vi "Init.vi"(8 "error in (no error)":errorcluster, 11 "Data in":refnum<class "Local Bus.lvclass">) -> (0 "error out":errorcluster, 3 "Data out":refnum<class "Local Bus.lvclass">)   [LabVIEW 2021, in "Local Bus.lvclass"]
uses:
  Local Bus.lvclass
  C:/TSA/Omni-Bus/Source/Omni-Bus/Bus Access/Bus_Access.lvclass
  Support/Type Counts.ctl
  Local Bus.lvclass/Local Bus.ctl
  Support/Type/Local Bus_Type.lvclass
  C:/Program Files (x86)/National Instruments/LabVIEW 2021/vi.lib/TSA/Abstract Data Classes/Abs_Types/Type/Abs_Type.lvclass
  Support/DBL/Local Bus_DBL.lvclass
  C:/Program Files (x86)/National Instruments/LabVIEW 2021/vi.lib/TSA/Abstract Data Classes/Abs_Types/Value/Abs_Value.lvclass
  Support/SGL/Local Bus_SGL.lvclass
  Support/EXT/Local Bus_EXT.lvclass
  Support/Bool/Local Bus_Boolean.lvclass
  Support/STR/Local Bus_String.lvclass
  Support/Variant/Local Bus_Variant.lvclass
  Support/WFM/Local Bus_Waveform.lvclass
  Support/Time/Local Bus_Time.lvclass
  Support/U8/Local Bus_U8.lvclass
  Support/U16/Local Bus_U16.lvclass
  Support/U32/Local Bus_U32.lvclass
  Support/U64/Local Bus_U64.lvclass
  Support/I8/Local Bus_I8.lvclass
  Support/I16/Local Bus_I16.lvclass
  Support/I32/Local Bus_I32.lvclass
  Support/I64/Local Bus_I64.lvclass
  Support/CSGL/Local Bus_CSGL.lvclass
  Support/CDBL/Local Bus_CDBL.lvclass
  Support/CEXT/Local Bus_CEXT.lvclass
  Omni-Bus/Bus Access/Bus_Access.lvclass/Bus_Access.ctl
  Properties/Read Tag Types.vi
  Properties/Read Initial Values.vi
  Omni-Bus/Bus Access/Properties/Write Values.vi
  <vilib>/TSA/Abstract Data Classes/Abs_Types/Value/Abs_Value.lvclass
  <vilib>/Utility/error.llb/Error Cluster From Error Code.vi
  <vilib>/ErrorRing/Error Ring.xnode
  Omni-Bus/Bus Access/Bus_Access.lvclass
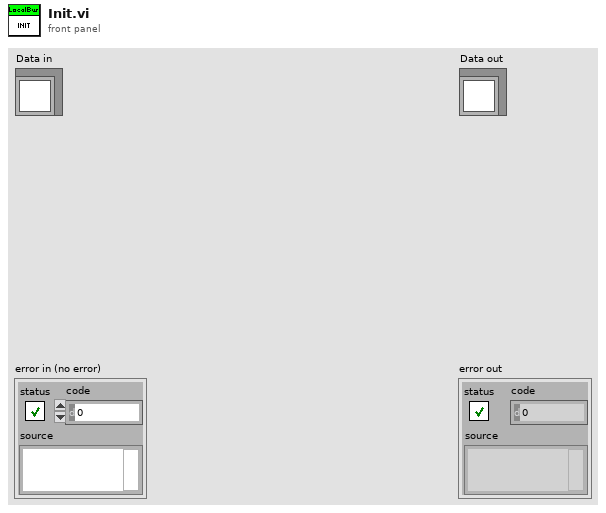
[diagram p1: front panel]
types:
  T1 = typedef "Local Bus.lvclass/Type Counts.ctl" = cluster{"Boolean":i32, "String":i32, "DBL":i32, "SGL":i32, "EXT":i32, "U8":i32, "U16":i32, "U32":i32, "U64":i32, "I8":i32, "I16":i32, "I32":i32, "I64":i32, "CDBL":i32, "CSGL":i32, "CEXT":i32, "Time":i32, "Variant":i32, "Waveform":i32, "Object":i32}
  T2 = typedef "NI_Data Type.lvlib/Data Type.ctl" = enum8{"Invalid Type", "Void", "I8", "I16", "I32", "I64", "U8", "U16", "U32", "U64", "Single Float", "Double Float", "Extended Float", "Single Complex", "Double Complex", "Extended Complex", "Enum U8", "Enum U16", "Enum U32", "Enum U64", "Single Float With Unit", "Double Float With Unit", "Extended Float With Unit", "Single Complex with Unit", "Double Complex with Unit", "Extended Complex with Unit", "Boolean", "String", "Path", "Picture", "Tag", "Array", "Cluster", "Variant", "LV Variant", "Waveform", "Timestamp", "Digital Waveform", "Digital Data", "ExpressData", "Refnum", "External Data", "VI", "Poly VI", "LabVIEW Class Instance", "Fixed Point", "Set Collection", "Map Collection"}
  T3 = typedef "Local Bus.lvclass/Data Value References.ctl" = cluster{"Boolean":refnum<data-value>, "String":refnum<data-value>, "DBL":refnum<data-value>, "SGL":refnum<data-value>, "EXT":refnum<data-value>, "U8":refnum<data-value>, "U16":refnum<data-value>, "U32":refnum<data-value>, "U64":refnum<data-value>, "I8":refnum<data-value>, "I16":refnum<data-value>, "I32":refnum<data-value>, "I64":refnum<data-value>, "CDBL":refnum<data-value>, "CSGL":refnum<data-value>, "CEXT":refnum<data-value>, "Time":refnum<data-value>, "Variant":refnum<data-value>, "Waveform":refnum<data-value>, "Type":refnum<data-value>}
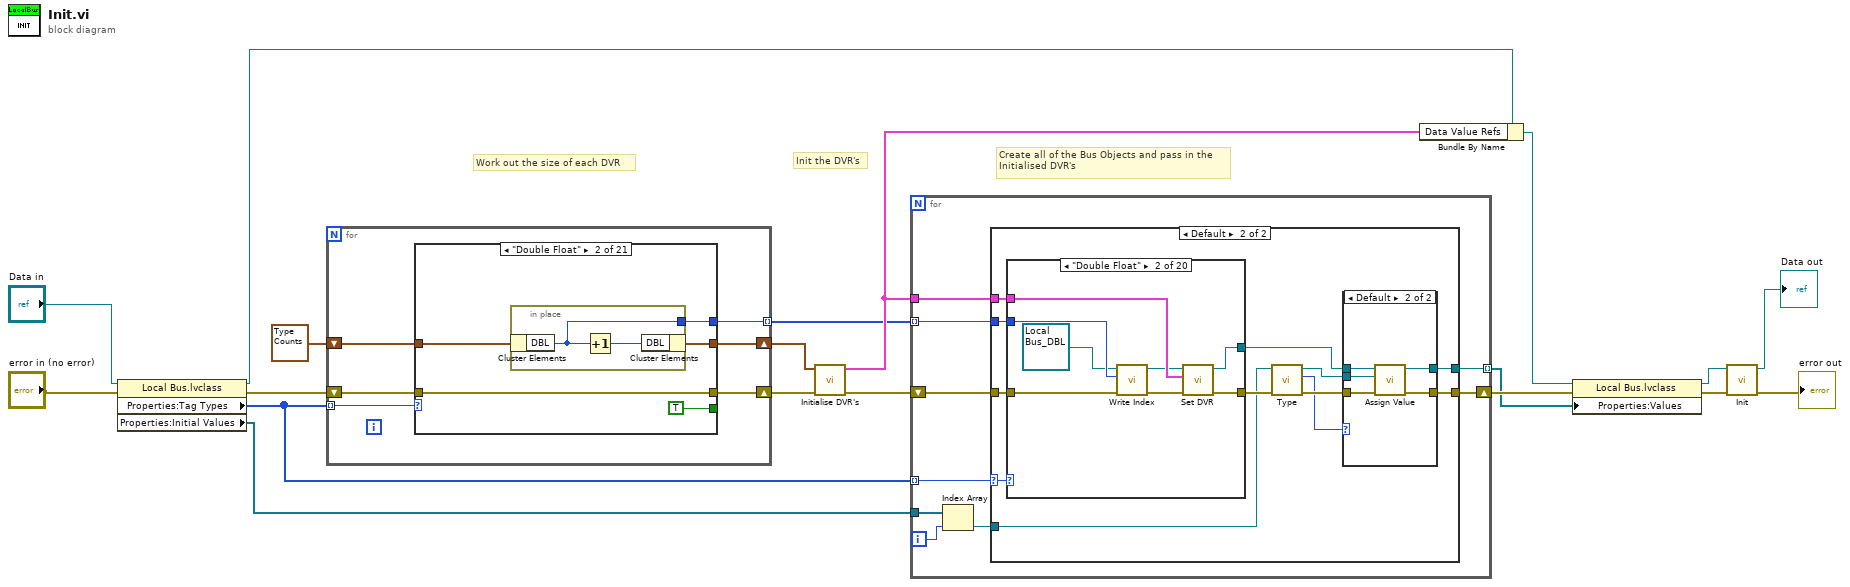
[diagram p0: block diagram]
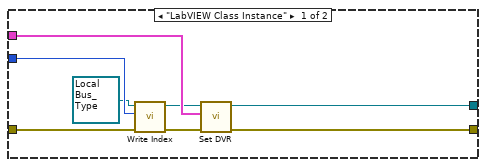
[diagram p2: hidden frame]
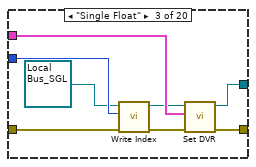
[diagram p5: hidden frame]
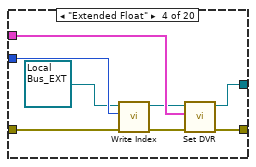
[diagram p6: hidden frame]
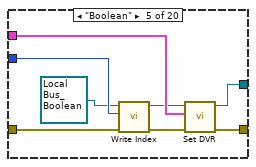
[diagram p7: hidden frame]
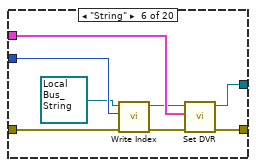
[diagram p8: hidden frame]
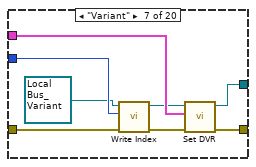
[diagram p9: hidden frame]
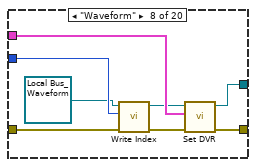
[diagram p10: hidden frame]
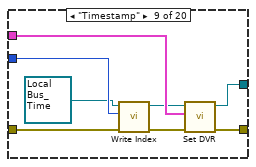
[diagram p11: hidden frame]
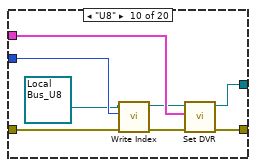
[diagram p12: hidden frame]
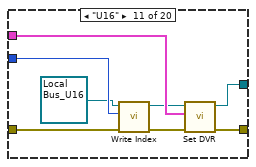
[diagram p13: hidden frame]
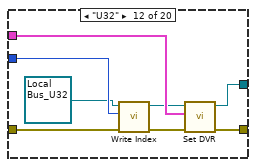
[diagram p14: hidden frame]
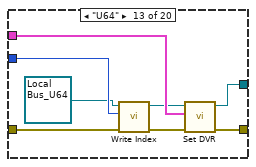
[diagram p15: hidden frame]
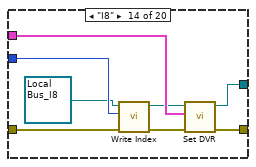
[diagram p16: hidden frame]
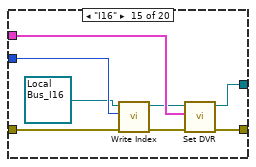
[diagram p17: hidden frame]
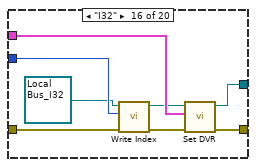
[diagram p18: hidden frame]
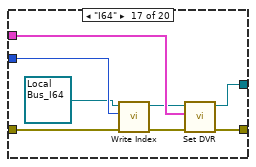
[diagram p19: hidden frame]
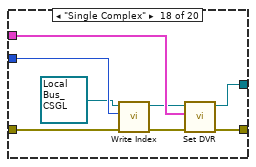
[diagram p20: hidden frame]
diagram:
  # "Create all of the Bus Objects and pass in the\nInitialised DVR's"
  # "Init the DVR's"
  # "Work out the size of each DVR"
  n1 = property class="Local Bus.lvclass"(reference="Data in", error in="error in (no error)") -> (reference out=w16:refnum<class "Local Bus.lvclass">, error out=w17:errorcluster, "Properties:Tag Types"=w6:T2[], "Properties:Initial Values"=w5:refnum<class "Abs_Value.lvclass">[])
  n2 = for {
    shift-right: [w22] -> w14
    shift-left: w17 -> [w25]
    shift-right: [w23] -> w13
    shift-left: T1 {"Boolean"=0, "String"=0, "DBL"=0, "SGL"=0, "EXT"=0, "U8"=0, "U16"=0, "U32"=0, "U64"=0, "I8"=0, "I16"=0, "I32"=0, "I64"=0, "CDBL"=0, "CSGL"=0, "CEXT"=0, "Time"=0, "Variant"=0, "Waveform"=0, "Object"=0} ("Type Counts") -> [w24]
    tunnel: [w21] -> w7 mode=indexing
    tunnel: w6 -> [w20] mode=indexing
    n3 = case shown="\"Double Float\"" w20 {
      tunnel: w25 -> [_ w38 w45 w52 w59 w66 w73 w80 w87 w94 w101 w108 w115 w122 w129 w136 w143 w150 w157 w164 w171]
      tunnel: w24 -> [w28 w37 w44 w51 w58 w65 w72 w79 w86 w93 w100 w107 w114 w121 w128 w135 w142 w149 w156 w163 w170]
      tunnel: [w28 w36 w43 w50 w57 w64 w71 w78 w85 w92 w99 w106 w113 w120 w127 w134 w141 w148 w155 w162 w169] -> w23
      tunnel: [w26 w38 w45 w52 w59 w66 w73 w80 w87 w94 w101 w108 w115 w122 w129 w136 w143 w150 w157 w164 w171] -> w22
      tunnel: [FALSE TRUE TRUE TRUE TRUE TRUE TRUE TRUE TRUE TRUE TRUE TRUE TRUE TRUE TRUE TRUE TRUE TRUE TRUE TRUE TRUE] -> _
      tunnel: [_ w34 w41 w48 w55 w62 w69 w76 w83 w90 w97 w104 w111 w118 w125 w132 w139 w146 w153 w160 w167] -> w21
      frame "Invalid Type", Default {
        n4 = xnode "Error Ring"() -> ("error out"=w26:errorcluster)
      }
      frame "Double Float" {
        n5 = in-place {
          in-place-border: [w39] -> w34
          n6 = in-place-cluster #1(w37) -> ("DBL"=w39:i32)
          n7 = Increment(x=w39) -> (x+1=w40:i32)
          n8 = in-place-cluster #1("DBL"=w40) -> (w36:T1)
        }
      }
      frame "Single Float" {
        n9 = in-place {
          in-place-border: [w46] -> w41
          n10 = in-place-cluster #2(w44) -> ("SGL"=w46:i32)
          n11 = Increment(x=w46) -> (x+1=w47:i32)
          n12 = in-place-cluster #2("SGL"=w47) -> (w43:T1)
        }
      }
      frame "Extended Float" {
        n13 = in-place {
          in-place-border: [w53] -> w48
          n14 = in-place-cluster #3(w51) -> ("EXT"=w53:i32)
          n15 = Increment(x=w53) -> (x+1=w54:i32)
          n16 = in-place-cluster #3("EXT"=w54) -> (w50:T1)
        }
      }
      frame "Boolean" {
        n17 = in-place {
          in-place-border: [w60] -> w55
          n18 = in-place-cluster #4(w58) -> ("Boolean"=w60:i32)
          n19 = Increment(x=w60) -> (x+1=w61:i32)
          n20 = in-place-cluster #4("Boolean"=w61) -> (w57:T1)
        }
      }
      frame "String" {
        n21 = in-place {
          in-place-border: [w67] -> w62
          n22 = in-place-cluster #5(w65) -> ("String"=w67:i32)
          n23 = Increment(x=w67) -> (x+1=w68:i32)
          n24 = in-place-cluster #5("String"=w68) -> (w64:T1)
        }
      }
      frame "Waveform" {
        n25 = in-place {
          in-place-border: [w74] -> w69
          n26 = in-place-cluster #6(w72) -> ("Waveform"=w74:i32)
          n27 = Increment(x=w74) -> (x+1=w75:i32)
          n28 = in-place-cluster #6("Waveform"=w75) -> (w71:T1)
        }
      }
      frame "Timestamp" {
        n29 = in-place {
          in-place-border: [w81] -> w76
          n30 = in-place-cluster #7(w79) -> ("Time"=w81:i32)
          n31 = Increment(x=w81) -> (x+1=w82:i32)
          n32 = in-place-cluster #7("Time"=w82) -> (w78:T1)
        }
      }
      frame "Variant" {
        n33 = in-place {
          in-place-border: [w88] -> w83
          n34 = in-place-cluster #8(w86) -> ("Variant"=w88:i32)
          n35 = Increment(x=w88) -> (x+1=w89:i32)
          n36 = in-place-cluster #8("Variant"=w89) -> (w85:T1)
        }
      }
      frame "LabVIEW Class Instance" {
        n37 = in-place {
          in-place-border: [w95] -> w90
          n38 = in-place-cluster #9(w93) -> ("Object"=w95:i32)
          n39 = Increment(x=w95) -> (x+1=w96:i32)
          n40 = in-place-cluster #9("Object"=w96) -> (w92:T1)
        }
      }
      frame "U8" {
        n41 = in-place {
          in-place-border: [w102] -> w97
          n42 = in-place-cluster #10(w100) -> ("U8"=w102:i32)
          n43 = Increment(x=w102) -> (x+1=w103:i32)
          n44 = in-place-cluster #10("U8"=w103) -> (w99:T1)
        }
      }
      frame "U16" {
        n45 = in-place {
          in-place-border: [w109] -> w104
          n46 = in-place-cluster #11(w107) -> ("U16"=w109:i32)
          n47 = Increment(x=w109) -> (x+1=w110:i32)
          n48 = in-place-cluster #11("U16"=w110) -> (w106:T1)
        }
      }
      frame "U32" {
        n49 = in-place {
          in-place-border: [w116] -> w111
          n50 = in-place-cluster #12(w114) -> ("U32"=w116:i32)
          n51 = Increment(x=w116) -> (x+1=w117:i32)
          n52 = in-place-cluster #12("U32"=w117) -> (w113:T1)
        }
      }
      frame "U64" {
        n53 = in-place {
          in-place-border: [w123] -> w118
          n54 = in-place-cluster #13(w121) -> ("U64"=w123:i32)
          n55 = Increment(x=w123) -> (x+1=w124:i32)
          n56 = in-place-cluster #13("U64"=w124) -> (w120:T1)
        }
      }
      frame "I8" {
        n57 = in-place {
          in-place-border: [w130] -> w125
          n58 = in-place-cluster #14(w128) -> ("I8"=w130:i32)
          n59 = Increment(x=w130) -> (x+1=w131:i32)
          n60 = in-place-cluster #14("I8"=w131) -> (w127:T1)
        }
      }
      frame "I16" {
        n61 = in-place {
          in-place-border: [w137] -> w132
          n62 = in-place-cluster #15(w135) -> ("I16"=w137:i32)
          n63 = Increment(x=w137) -> (x+1=w138:i32)
          n64 = in-place-cluster #15("I16"=w138) -> (w134:T1)
        }
      }
      frame "I32" {
        n65 = in-place {
          in-place-border: [w144] -> w139
          n66 = in-place-cluster #16(w142) -> ("I32"=w144:i32)
          n67 = Increment(x=w144) -> (x+1=w145:i32)
          n68 = in-place-cluster #16("I32"=w145) -> (w141:T1)
        }
      }
      frame "I64" {
        n69 = in-place {
          in-place-border: [w151] -> w146
          n70 = in-place-cluster #17(w149) -> ("I64"=w151:i32)
          n71 = Increment(x=w151) -> (x+1=w152:i32)
          n72 = in-place-cluster #17("I64"=w152) -> (w148:T1)
        }
      }
      frame "Single Complex" {
        n73 = in-place {
          in-place-border: [w158] -> w153
          n74 = in-place-cluster #18(w156) -> ("CSGL"=w158:i32)
          n75 = Increment(x=w158) -> (x+1=w159:i32)
          n76 = in-place-cluster #18("CSGL"=w159) -> (w155:T1)
        }
      }
      frame "Double Complex" {
        n77 = in-place {
          in-place-border: [w165] -> w160
          n78 = in-place-cluster #19(w163) -> ("CDBL"=w165:i32)
          n79 = Increment(x=w165) -> (x+1=w166:i32)
          n80 = in-place-cluster #19("CDBL"=w166) -> (w162:T1)
        }
      }
      frame "Extended Complex" {
        n81 = in-place {
          in-place-border: [w172] -> w167
          n82 = in-place-cluster #20(w170) -> ("CEXT"=w172:i32)
          n83 = Increment(x=w172) -> (x+1=w173:i32)
          n84 = in-place-cluster #20("CEXT"=w173) -> (w169:T1)
        }
      }
    }
  }
  n85 = call "Initialise DVR's.vi"("error in (no error)"=w14, "Type Counts"=w13) -> ("error out"=w12:errorcluster, "Data Value References"=w8:T3)  [unwired: 8 in]
  n86 = for {
    tunnel: w8 -> [w182]
    tunnel: [w178] -> w10 mode=indexing
    shift-right: [w177] -> w11
    shift-left: w12 -> [w181]
    tunnel: w7 -> [w180] mode=indexing
    tunnel: w6 -> [w179] mode=indexing
    tunnel: w5 -> [w176]
    i -> [w175]
    n87 = Index Array(array=w176, index=w175) -> (element=w174:refnum<class "Abs_Value.lvclass">)
    n88 = case shown="Default" w179 {
      selector: w179 -> [_ w199]
      tunnel: w182 -> [w190 w202]
      tunnel: w181 -> [w189 w201]
      tunnel: w180 -> [w188 w200]
      tunnel: [w184 w196] -> w178
      tunnel: [w183 w197] -> w177
      tunnel: w174 -> [_ w194]
      frame "LabVIEW Class Instance" {
        n89 = call-dynamic "Write Index.vi"("error in (no error)"=w189, "Index"=w188, "Local Bus_Access in"=refnum<class "Local Bus_Type.lvclass"> refnum ("Local Bus_Type.lvclass")) -> ("error out"=w187:errorcluster, "Local Bus_Access out"=w186:refnum<class "Local Bus_Type.lvclass">)  [unwired: 7 in]
        n90 = call-dynamic "Set DVR.vi"("error in (no error)"=w187, "Type Counts"=w190, "Local Bus_DBL in"=w186) -> ("error out"=w183:errorcluster, "Local Bus_DBL out"=w184:refnum<class "Local Bus_Type.lvclass">)  [unwired: 7 in]
      }
      frame Default {
        n91 = case shown="\"Double Float\"" w199 {
          tunnel: [w210 w218 w226 w234 w242 w250 w258 w266 w274 w282 w290 w298 w306 w314 w322 w330 w338 w346 w354 w362] -> w195
          tunnel: w202 -> [_ w217 w225 w233 w241 w249 w257 w265 w273 w281 w289 w297 w305 w313 w321 w329 w337 w345 w353 w361]
          tunnel: [_ w216 w224 w232 w240 w248 w256 w264 w272 w280 w288 w296 w304 w312 w320 w328 w336 w344 w352 w360] -> w198
          tunnel: w201 -> [w210 w215 w223 w231 w239 w247 w255 w263 w271 w279 w287 w295 w303 w311 w319 w327 w335 w343 w351 w359]
          tunnel: w200 -> [_ w212 w220 w228 w236 w244 w252 w260 w268 w276 w284 w292 w300 w308 w316 w324 w332 w340 w348 w356]
          frame "Invalid Type", Default {
          }
          frame "Double Float" {
            n92 = call-dynamic "Write Index.vi"("error in (no error)"=w215, "Index"=w212, "Local Bus_Access in"=refnum<class "Local Bus_DBL.lvclass"> refnum ("Local Bus_DBL.lvclass")) -> ("error out"=w214:errorcluster, "Local Bus_Access out"=w213:refnum<class "Local Bus_DBL.lvclass">)  [unwired: 7 in]
            n93 = call-dynamic "Set DVR.vi"("error in (no error)"=w214, "Type Counts"=w217, "Local Bus_DBL in"=w213) -> ("error out"=w218:errorcluster, "Local Bus_DBL out"=w216:refnum<class "Local Bus_DBL.lvclass">)  [unwired: 7 in]
          }
          frame "Single Float" {
            n94 = call-dynamic "Write Index.vi"("error in (no error)"=w223, "Index"=w220, "Local Bus_Access in"=refnum<class "Local Bus_SGL.lvclass"> refnum ("Local Bus_SGL.lvclass")) -> ("error out"=w222:errorcluster, "Local Bus_Access out"=w221:refnum<class "Local Bus_SGL.lvclass">)  [unwired: 7 in]
            n95 = call-dynamic "Set DVR.vi"("error in (no error)"=w222, "Type Counts"=w225, "Local Bus_DBL in"=w221) -> ("error out"=w226:errorcluster, "Local Bus_DBL out"=w224:refnum<class "Local Bus_SGL.lvclass">)  [unwired: 7 in]
          }
          frame "Extended Float" {
            n96 = call-dynamic "Write Index.vi"("error in (no error)"=w231, "Index"=w228, "Local Bus_Access in"=refnum<class "Local Bus_EXT.lvclass"> refnum ("Local Bus_EXT.lvclass")) -> ("error out"=w230:errorcluster, "Local Bus_Access out"=w229:refnum<class "Local Bus_EXT.lvclass">)  [unwired: 7 in]
            n97 = call-dynamic "Set DVR.vi"("error in (no error)"=w230, "Type Counts"=w233, "Local Bus_DBL in"=w229) -> ("error out"=w234:errorcluster, "Local Bus_DBL out"=w232:refnum<class "Local Bus_EXT.lvclass">)  [unwired: 7 in]
          }
          frame "Boolean" {
            n98 = call-dynamic "Write Index.vi"("error in (no error)"=w239, "Index"=w236, "Local Bus_Access in"=refnum<class "Local Bus_Boolean.lvclass"> refnum ("Local Bus_Boolean.lvclass")) -> ("error out"=w238:errorcluster, "Local Bus_Access out"=w237:refnum<class "Local Bus_Boolean.lvclass">)  [unwired: 7 in]
            n99 = call-dynamic "Set DVR.vi"("error in (no error)"=w238, "Type Counts"=w241, "Local Bus_DBL in"=w237) -> ("error out"=w242:errorcluster, "Local Bus_DBL out"=w240:refnum<class "Local Bus_Boolean.lvclass">)  [unwired: 7 in]
          }
          frame "String" {
            n100 = call-dynamic "Write Index.vi"("error in (no error)"=w247, "Index"=w244, "Local Bus_Access in"=refnum<class "Local Bus_String.lvclass"> refnum ("Local Bus_String.lvclass")) -> ("error out"=w246:errorcluster, "Local Bus_Access out"=w245:refnum<class "Local Bus_String.lvclass">)  [unwired: 7 in]
            n101 = call-dynamic "Set DVR.vi"("error in (no error)"=w246, "Type Counts"=w249, "Local Bus_DBL in"=w245) -> ("error out"=w250:errorcluster, "Local Bus_DBL out"=w248:refnum<class "Local Bus_String.lvclass">)  [unwired: 7 in]
          }
          frame "Variant" {
            n102 = call-dynamic "Write Index.vi"("error in (no error)"=w255, "Index"=w252, "Local Bus_Access in"=refnum<class "Local Bus_Variant.lvclass"> refnum ("Local Bus_Variant.lvclass")) -> ("error out"=w254:errorcluster, "Local Bus_Access out"=w253:refnum<class "Local Bus_Variant.lvclass">)  [unwired: 7 in]
            n103 = call-dynamic "Set DVR.vi"("error in (no error)"=w254, "Type Counts"=w257, "Local Bus_DBL in"=w253) -> ("error out"=w258:errorcluster, "Local Bus_DBL out"=w256:refnum<class "Local Bus_Variant.lvclass">)  [unwired: 7 in]
          }
          frame "Waveform" {
            n104 = call-dynamic "Write Index.vi"("error in (no error)"=w263, "Index"=w260, "Local Bus_Access in"=refnum<class "Local Bus_Waveform.lvclass"> refnum ("Local Bus_Waveform.lvclass")) -> ("error out"=w262:errorcluster, "Local Bus_Access out"=w261:refnum<class "Local Bus_Waveform.lvclass">)  [unwired: 7 in]
            n105 = call-dynamic "Set DVR.vi"("error in (no error)"=w262, "Type Counts"=w265, "Local Bus_DBL in"=w261) -> ("error out"=w266:errorcluster, "Local Bus_DBL out"=w264:refnum<class "Local Bus_Waveform.lvclass">)  [unwired: 7 in]
          }
          frame "Timestamp" {
            n106 = call-dynamic "Write Index.vi"("error in (no error)"=w271, "Index"=w268, "Local Bus_Access in"=refnum<class "Local Bus_Time.lvclass"> refnum ("Local Bus_Time.lvclass")) -> ("error out"=w270:errorcluster, "Local Bus_Access out"=w269:refnum<class "Local Bus_Time.lvclass">)  [unwired: 7 in]
            n107 = call-dynamic "Set DVR.vi"("error in (no error)"=w270, "Type Counts"=w273, "Local Bus_DBL in"=w269) -> ("error out"=w274:errorcluster, "Local Bus_DBL out"=w272:refnum<class "Local Bus_Time.lvclass">)  [unwired: 7 in]
          }
          frame "U8" {
            n108 = call-dynamic "Write Index.vi"("error in (no error)"=w279, "Index"=w276, "Local Bus_Access in"=refnum<class "Local Bus_U8.lvclass"> refnum ("Local Bus_U8.lvclass")) -> ("error out"=w278:errorcluster, "Local Bus_Access out"=w277:refnum<class "Local Bus_U8.lvclass">)  [unwired: 7 in]
            n109 = call-dynamic "Set DVR.vi"("error in (no error)"=w278, "Type Counts"=w281, "Local Bus_DBL in"=w277) -> ("error out"=w282:errorcluster, "Local Bus_DBL out"=w280:refnum<class "Local Bus_U8.lvclass">)  [unwired: 7 in]
          }
          frame "U16" {
            n110 = call-dynamic "Write Index.vi"("error in (no error)"=w287, "Index"=w284, "Local Bus_Access in"=refnum<class "Local Bus_U16.lvclass"> refnum ("Local Bus_U16.lvclass")) -> ("error out"=w286:errorcluster, "Local Bus_Access out"=w285:refnum<class "Local Bus_U16.lvclass">)  [unwired: 7 in]
            n111 = call-dynamic "Set DVR.vi"("error in (no error)"=w286, "Type Counts"=w289, "Local Bus_DBL in"=w285) -> ("error out"=w290:errorcluster, "Local Bus_DBL out"=w288:refnum<class "Local Bus_U16.lvclass">)  [unwired: 7 in]
          }
          frame "U32" {
            n112 = call-dynamic "Write Index.vi"("error in (no error)"=w295, "Index"=w292, "Local Bus_Access in"=refnum<class "Local Bus_U32.lvclass"> refnum ("Local Bus_U32.lvclass")) -> ("error out"=w294:errorcluster, "Local Bus_Access out"=w293:refnum<class "Local Bus_U32.lvclass">)  [unwired: 7 in]
            n113 = call-dynamic "Set DVR.vi"("error in (no error)"=w294, "Type Counts"=w297, "Local Bus_DBL in"=w293) -> ("error out"=w298:errorcluster, "Local Bus_DBL out"=w296:refnum<class "Local Bus_U32.lvclass">)  [unwired: 7 in]
          }
          frame "U64" {
            n114 = call-dynamic "Write Index.vi"("error in (no error)"=w303, "Index"=w300, "Local Bus_Access in"=refnum<class "Local Bus_U64.lvclass"> refnum ("Local Bus_U64.lvclass")) -> ("error out"=w302:errorcluster, "Local Bus_Access out"=w301:refnum<class "Local Bus_U64.lvclass">)  [unwired: 7 in]
            n115 = call-dynamic "Set DVR.vi"("error in (no error)"=w302, "Type Counts"=w305, "Local Bus_DBL in"=w301) -> ("error out"=w306:errorcluster, "Local Bus_DBL out"=w304:refnum<class "Local Bus_U64.lvclass">)  [unwired: 7 in]
          }
          frame "I8" {
            n116 = call-dynamic "Write Index.vi"("error in (no error)"=w311, "Index"=w308, "Local Bus_Access in"=refnum<class "Local Bus_I8.lvclass"> refnum ("Local Bus_I8.lvclass")) -> ("error out"=w310:errorcluster, "Local Bus_Access out"=w309:refnum<class "Local Bus_I8.lvclass">)  [unwired: 7 in]
            n117 = call-dynamic "Set DVR.vi"("error in (no error)"=w310, "Type Counts"=w313, "Local Bus_DBL in"=w309) -> ("error out"=w314:errorcluster, "Local Bus_DBL out"=w312:refnum<class "Local Bus_I8.lvclass">)  [unwired: 7 in]
          }
          frame "I16" {
            n118 = call-dynamic "Write Index.vi"("error in (no error)"=w319, "Index"=w316, "Local Bus_Access in"=refnum<class "Local Bus_I16.lvclass"> refnum ("Local Bus_I16.lvclass")) -> ("error out"=w318:errorcluster, "Local Bus_Access out"=w317:refnum<class "Local Bus_I16.lvclass">)  [unwired: 7 in]
            n119 = call-dynamic "Set DVR.vi"("error in (no error)"=w318, "Type Counts"=w321, "Local Bus_DBL in"=w317) -> ("error out"=w322:errorcluster, "Local Bus_DBL out"=w320:refnum<class "Local Bus_I16.lvclass">)  [unwired: 7 in]
          }
          frame "I32" {
            n120 = call-dynamic "Write Index.vi"("error in (no error)"=w327, "Index"=w324, "Local Bus_Access in"=refnum<class "Local Bus_I32.lvclass"> refnum ("Local Bus_I32.lvclass")) -> ("error out"=w326:errorcluster, "Local Bus_Access out"=w325:refnum<class "Local Bus_I32.lvclass">)  [unwired: 7 in]
            n121 = call-dynamic "Set DVR.vi"("error in (no error)"=w326, "Type Counts"=w329, "Local Bus_DBL in"=w325) -> ("error out"=w330:errorcluster, "Local Bus_DBL out"=w328:refnum<class "Local Bus_I32.lvclass">)  [unwired: 7 in]
          }
          frame "I64" {
            n122 = call-dynamic "Write Index.vi"("error in (no error)"=w335, "Index"=w332, "Local Bus_Access in"=refnum<class "Local Bus_I64.lvclass"> refnum ("Local Bus_I64.lvclass")) -> ("error out"=w334:errorcluster, "Local Bus_Access out"=w333:refnum<class "Local Bus_I64.lvclass">)  [unwired: 7 in]
            n123 = call-dynamic "Set DVR.vi"("error in (no error)"=w334, "Type Counts"=w337, "Local Bus_DBL in"=w333) -> ("error out"=w338:errorcluster, "Local Bus_DBL out"=w336:refnum<class "Local Bus_I64.lvclass">)  [unwired: 7 in]
          }
          frame "Single Complex" {
            n124 = call-dynamic "Write Index.vi"("error in (no error)"=w343, "Index"=w340, "Local Bus_Access in"=refnum<class "Local Bus_CSGL.lvclass"> refnum ("Local Bus_CSGL.lvclass")) -> ("error out"=w342:errorcluster, "Local Bus_Access out"=w341:refnum<class "Local Bus_CSGL.lvclass">)  [unwired: 7 in]
            n125 = call-dynamic "Set DVR.vi"("error in (no error)"=w342, "Type Counts"=w345, "Local Bus_DBL in"=w341) -> ("error out"=w346:errorcluster, "Local Bus_DBL out"=w344:refnum<class "Local Bus_CSGL.lvclass">)  [unwired: 7 in]
          }
          frame "Double Complex" {
            n126 = call-dynamic "Write Index.vi"("error in (no error)"=w351, "Index"=w348, "Local Bus_Access in"=refnum<class "Local Bus_CDBL.lvclass"> refnum ("Local Bus_CDBL.lvclass")) -> ("error out"=w350:errorcluster, "Local Bus_Access out"=w349:refnum<class "Local Bus_CDBL.lvclass">)  [unwired: 7 in]
            n127 = call-dynamic "Set DVR.vi"("error in (no error)"=w350, "Type Counts"=w353, "Local Bus_DBL in"=w349) -> ("error out"=w354:errorcluster, "Local Bus_DBL out"=w352:refnum<class "Local Bus_CDBL.lvclass">)  [unwired: 7 in]
          }
          frame "Extended Complex" {
            n128 = call-dynamic "Write Index.vi"("error in (no error)"=w359, "Index"=w356, "Local Bus_Access in"=refnum<class "Local Bus_CEXT.lvclass"> refnum ("Local Bus_CEXT.lvclass")) -> ("error out"=w358:errorcluster, "Local Bus_Access out"=w357:refnum<class "Local Bus_CEXT.lvclass">)  [unwired: 7 in]
            n129 = call-dynamic "Set DVR.vi"("error in (no error)"=w358, "Type Counts"=w361, "Local Bus_DBL in"=w357) -> ("error out"=w362:errorcluster, "Local Bus_DBL out"=w360:refnum<class "Local Bus_CEXT.lvclass">)  [unwired: 7 in]
          }
        }
        n130 = call-dynamic "Type.vi"("error in (no error)"=w195, "Element in"=w194) -> ("error out"=w193:errorcluster, "Type"=w191:T2, "Element out"=w192:refnum<class "Abs_Value.lvclass">)  [unwired: 7 in]
        n131 = case shown="Default" w191 {
          tunnel: w198 -> [w203 w209]
          tunnel: [w204 w208] -> w197
          tunnel: [w203 w207] -> w196
          tunnel: w193 -> [w204 w206]
          tunnel: w192 -> [_ w205]
          frame "Invalid Type" {
          }
          frame Default {
            n132 = call-dynamic "Assign Value.vi"("error in (no error)"=w206, "Assigned Value"=w205, "Abs_Value in"=w209) -> ("error out"=w208:errorcluster, "Abs_Value out"=w207:refnum<class "Abs_Value.lvclass">)  [unwired: 7 in]
          }
        }
      }
    }
  }
  n133 = Bundle By Name(cluster=w16, "Data Value Refs"=w8) -> (w9:refnum<class "Local Bus.lvclass">)
  n134 = property class="Local Bus.lvclass"(reference=w9, error in=w11, "Properties:Values"=w10) -> (reference out=w2:refnum<class "Local Bus.lvclass">, error out=w4:errorcluster)
  n135 = call-parent "Init.vi"("error in (no error)"=w4, "Data in"=w2) -> ("error out"=→"error out":errorcluster, "Data out"=→"Data out":refnum<class "Local Bus.lvclass">)  [unwired: 8 in]
